vi "SwerveOdometry_UpdateX.vi"(8 "module Positions":T6[](array[typedef]) {"Angle"."SIN" format="%13.4f"; "Angle"."COS" format="%13.4f"; "Angle"."VALUE" format="%13.4f"}, 9 "gyroAngle":T5={"VALUE"=0.0, "COS"=1.0, "SIN"=0.0} {"SIN" format="%13.4f"; "COS" format="%13.4f"; "VALUE" format="%13.4f"}, 10 "in SWERVE_DRIVE_ODOMETRY":T8={"POSE"={"TRANSLATION"={"X"=0.0, "Y"=0.0}, "ROTATION"={"VALUE"=0.0, "COS"=1.0, "SIN"=0.0}}, "GyroOffset"={"VALUE"=0.0, "COS"=1.0, "SIN"=0.0}, "PreviousAngle"={"VALUE"=0.0, "COS"=1.0, "SIN"=0.0}, "PrevModulePositions"=[], "NumModules"=0} {"PrevModulePositions"."Angle"."SIN" format="%13.4f"; "PrevModulePositions"."Angle"."COS" format="%13.4f"; "PrevModulePositions"."Angle"."VALUE" format="%13.4f"; "PreviousAngle"."SIN" format="%13.4f"; "PreviousAngle"."COS" format="%13.4f"; "PreviousAngle"."VALUE" format="%13.4f"; "GyroOffset"."SIN" format="%13.4f"; "GyroOffset"."COS" format="%13.4f"; "GyroOffset"."VALUE" format="%13.4f"; "POSE"."ROTATION"."SIN" format="%13.4f"; "POSE"."ROTATION"."COS" format="%13.4f"; "POSE"."ROTATION"."VALUE" format="%13.4f"; "POSE"."TRANSLATION"."Y" format="%14.3f"; "POSE"."TRANSLATION"."X" format="%14.3f"}, 11 "SWERVE_DRIVE_KINEMATICS":T1 {"SavedModuleStates"."Angle"."SIN" format="%13.4f"; "SavedModuleStates"."Angle"."COS" format="%13.4f"; "SavedModuleStates"."Angle"."VALUE" format="%13.4f"; "PrevCoR"."Y" format="%14.3f"; "PrevCoR"."X" format="%14.3f"; "Modules"."Y" format="%14.3f"; "Modules"."X" format="%14.3f"}) -> (0 "Error":bool, 1 "robot POSE":T7={"TRANSLATION"={"X"=0.0, "Y"=0.0}, "ROTATION"={"VALUE"=0.0, "COS"=1.0, "SIN"=0.0}} {"ROTATION"."SIN" format="%13.4f"; "ROTATION"."COS" format="%13.4f"; "ROTATION"."VALUE" format="%13.4f"; "TRANSLATION"."Y" format="%14.3f"; "TRANSLATION"."X" format="%14.3f"}, 3 "out SWERVE_DRIVE_ODOMETRY":T8={"POSE"={"TRANSLATION"={"X"=0.0, "Y"=0.0}, "ROTATION"={"VALUE"=0.0, "COS"=1.0, "SIN"=0.0}}, "GyroOffset"={"VALUE"=0.0, "COS"=1.0, "SIN"=0.0}, "PreviousAngle"={"VALUE"=0.0, "COS"=1.0, "SIN"=0.0}, "PrevModulePositions"=[], "NumModules"=0} {"PrevModulePositions"."Angle"."SIN" format="%13.4f"; "PrevModulePositions"."Angle"."COS" format="%13.4f"; "PrevModulePositions"."Angle"."VALUE" format="%13.4f"; "PreviousAngle"."SIN" format="%13.4f"; "PreviousAngle"."COS" format="%13.4f"; "PreviousAngle"."VALUE" format="%13.4f"; "GyroOffset"."SIN" format="%13.4f"; "GyroOffset"."COS" format="%13.4f"; "GyroOffset"."VALUE" format="%13.4f"; "POSE"."ROTATION"."SIN" format="%13.4f"; "POSE"."ROTATION"."COS" format="%13.4f"; "POSE"."ROTATION"."VALUE" format="%13.4f"; "POSE"."TRANSLATION"."Y" format="%14.3f"; "POSE"."TRANSLATION"."X" format="%14.3f"})   [LabVIEW 2019, in "Trajectory_Library.lvlib"]
doc: "Updates the robot's position on the field using forward kinematics and integration of the pose over time. This method takes in the current time as a parameter to calculate period (difference between two timestamps). The period is used to calculate the change in distance from a velocity. Thisalso takes in an angle parameter which is used instead of the angular rate that is calculated from forward kinematics.\n\nParameters:\n - InSwerveDriveKinematics - The data structure \n - InSwerveDriveOdometry - This data structure \n - gyroAngle - The angle reported by the gyroscope.\n - modulePositions - The current positions (distances) of all swerve modules. Please provide the states in the same order in which you instantiated your SwerveDriveKinematics.\n\nReturns:\n - OutSwerveDriveOdometry - Updated data structure\n - The new pose of the robot.\n - Error -- TRUE if an error occured (number of modules doesn't match)"
uses:
  Trajectory_Library.lvlib
  TypeDef/TRANSLATION2D.ctl
  TypeDef/ROTATION2D.ctl
  TypeDef/POSE2D.ctl
  TypeDef/SWERVE_DRIVE_ODOMETRY.ctl
  TypeDef/SWERVE_DRIVE_MODULE_STATE.ctl
  <vilib>/Analysis/Matrix/Datatypes/RealMatrix.ctl
  <vilib>/Analysis/Matrix/NI_Matrix.lvlib
  TypeDef/SWERVE_DRIVE_KINEMATICS.ctl
  TypeDef/SWERVE_DRIVE_MODULE_POSITION.ctl
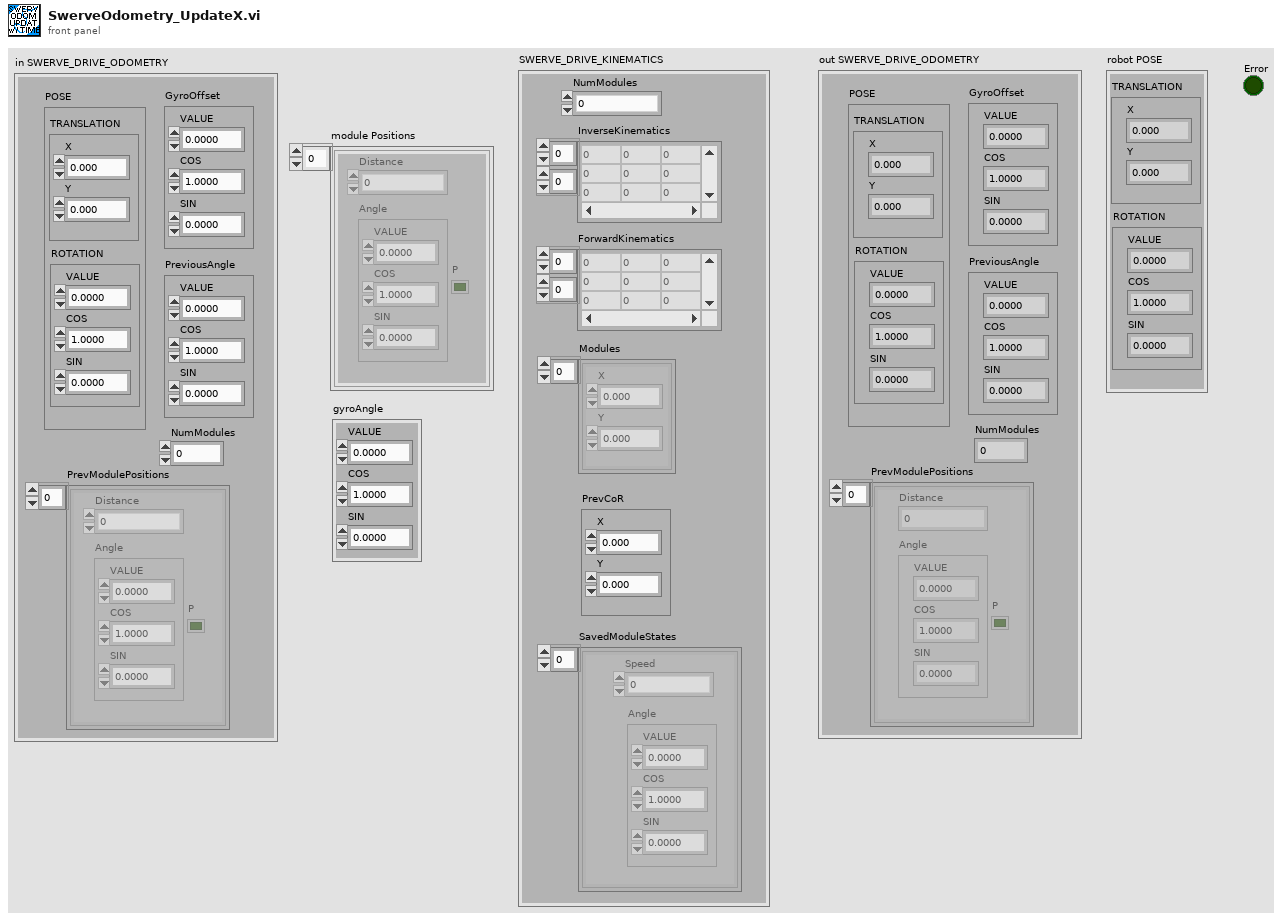
[diagram p1: front panel]
types:
  T1 = typedef "Trajectory_Library.lvlib/SWERVE_DRIVE_KINEMATICS.ctl" = cluster{"NumModules":i32, "InverseKinematics":T2, "ForwardKinematics":T2, "Modules":T3[], "PrevCoR":T3, "SavedModuleStates":T4[]}
  T2 = typedef "NI_Matrix.lvlib/RealMatrix.ctl" = dbl[][]
  T3 = typedef "Trajectory_Library.lvlib/TRANSLATION2D.ctl" = cluster{"X":dbl, "Y":dbl}
  T4 = typedef "Trajectory_Library.lvlib/SWERVE_DRIVE_MODULE_STATE.ctl" = cluster{"Speed":dbl, "Angle":T5}
  T5 = typedef "Trajectory_Library.lvlib/ROTATION2D.ctl" = cluster{"VALUE":dbl, "COS":dbl, "SIN":dbl}
  T6 = typedef "Trajectory_Library.lvlib/SWERVE_DRIVE_MODULE_POSITION.ctl" = cluster{"Distance":dbl, "Angle":T5, "P":bool}
  T7 = typedef "Trajectory_Library.lvlib/POSE2D.ctl" = cluster{"TRANSLATION":T3, "ROTATION":T5}
  T8 = typedef "Trajectory_Library.lvlib/SWERVE_DRIVE_ODOMETRY.ctl" = cluster{"POSE":T7, "GyroOffset":T5, "PreviousAngle":T5, "PrevModulePositions":T6[], "NumModules":i32}
  T9 = typedef "Trajectory_Library.lvlib/TWIST2D.ctl" = cluster{"dX":dbl, "dY":dbl, "dTHETA":dbl}
  T10 = typedef "WPILib_Math.lvlib/POSE2D.ctl" = cluster{"TRANSLATION":T11, "ROTATION":T12}
  T11 = typedef "WPILib_Math.lvlib/TRANSLATION2D.ctl" = cluster{"X":dbl, "Y":dbl}
  T12 = typedef "WPILib_Math.lvlib/ROTATION2D.ctl" = cluster{"VALUE":dbl, "COS":dbl, "SIN":dbl}
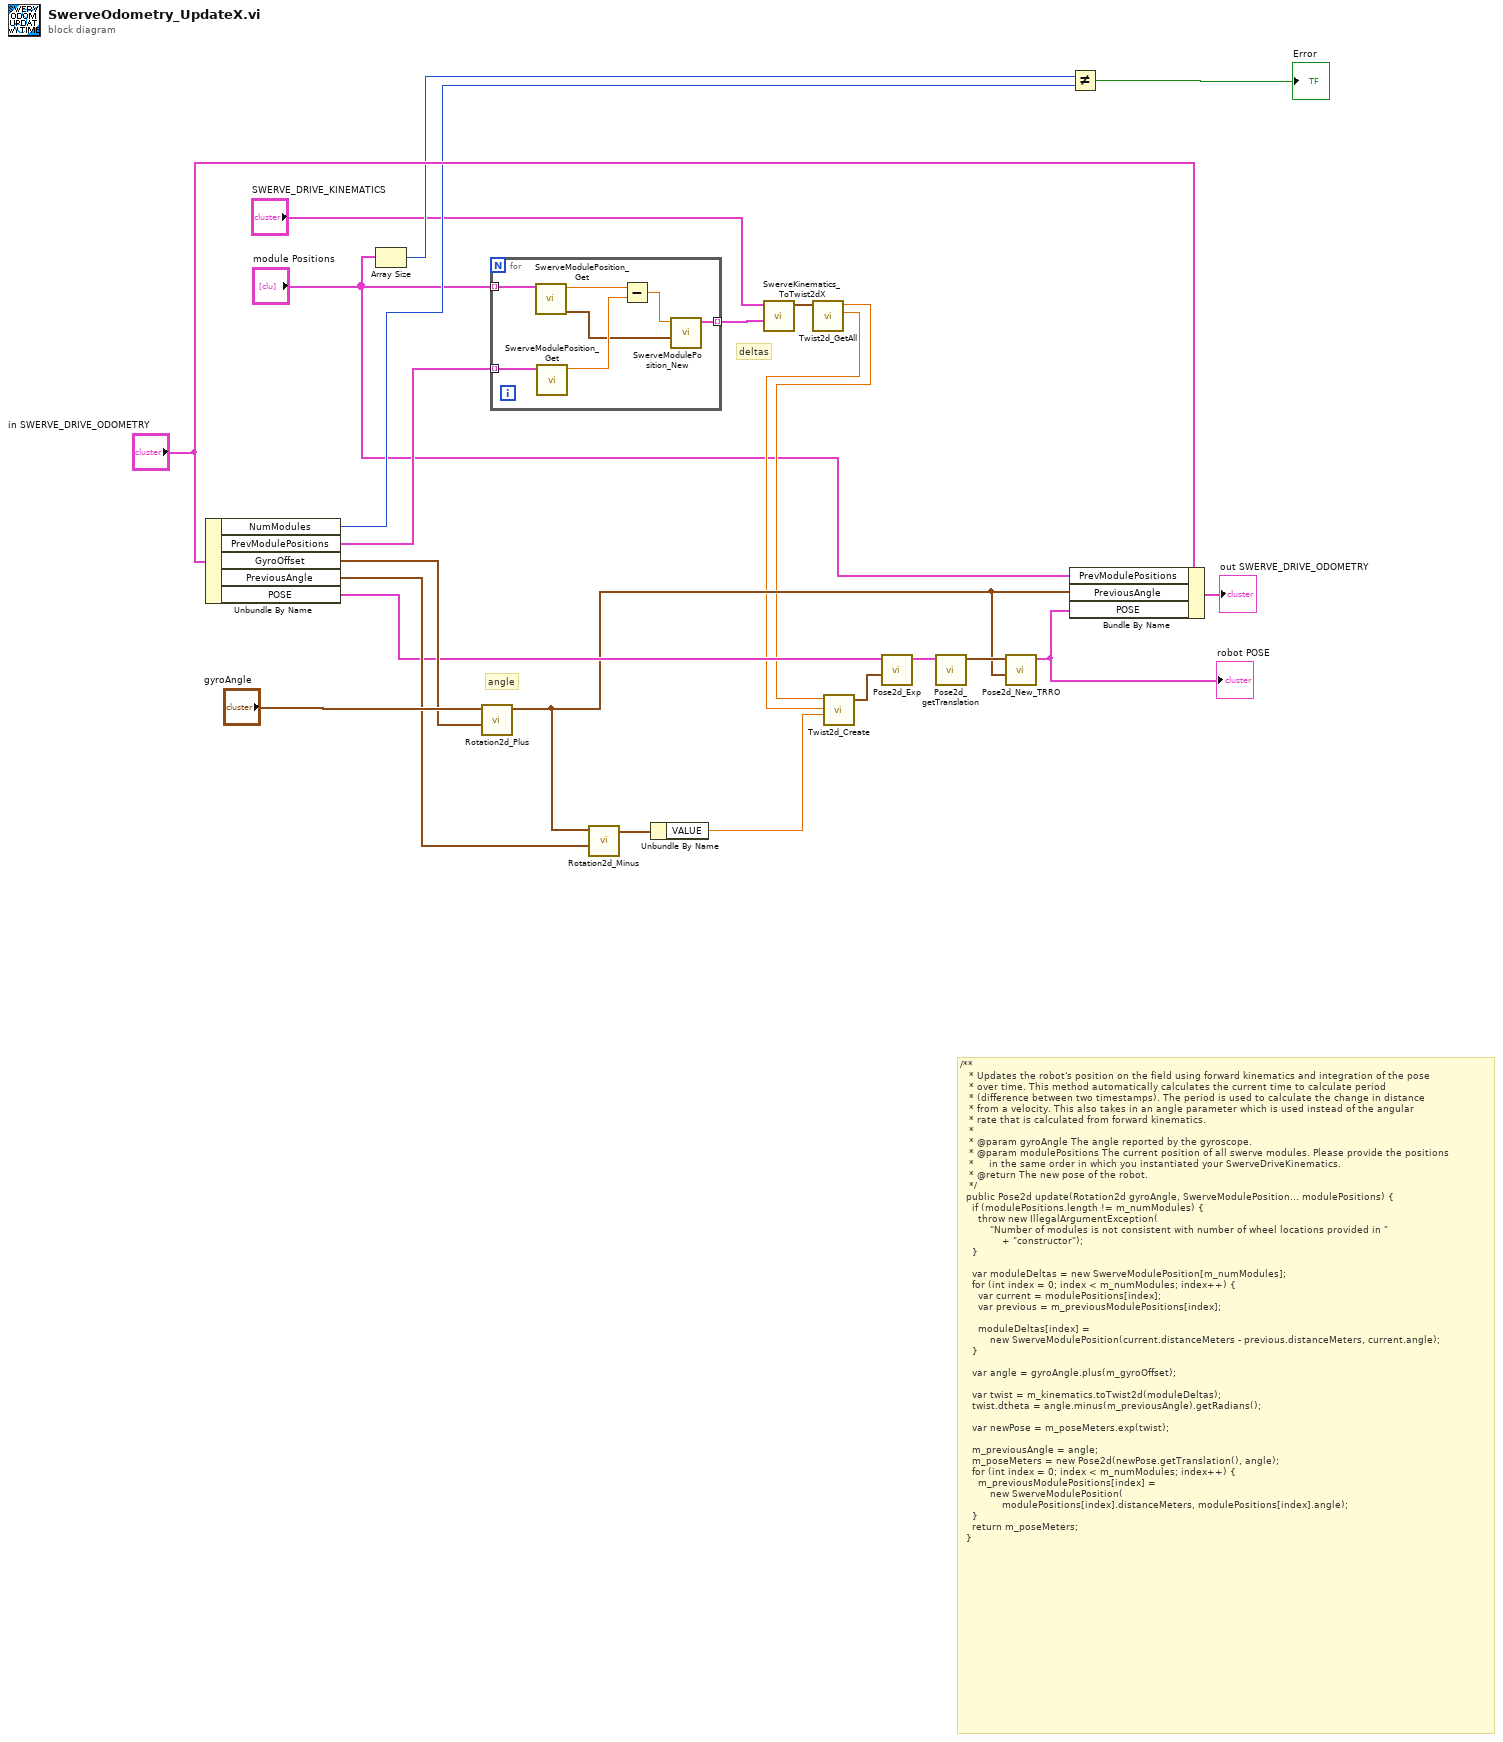
[diagram p0: block diagram]
diagram:
  # "deltas"
  # "/**\n   * Updates the robot's position on the field using forward kinematics and integration of the pose\n   * over time. This method automatically calculates the current time to calculate period\n   * (difference between two timestamps). The period is used to calculate the change in distance\n   * from a velocity. This also takes in an angle parameter which is used instead of the angular\n   * rate that is calculated from forward kinematics.\n   *\n   * @param gyroAngle The angle reported by the gyroscope.\n   * @param modulePositions The current position of all swerve modules. Please provide the positions\n   *     in the same order in which you instantiated your SwerveDriveKinematics.\n   * @return The new pose of the robot.\n   */\n  public Pose2d update(Rotation2d gyroAngle, SwerveModulePosition... modulePositions) {\n    if (modulePositions.length != m_numModules) {\n      throw new IllegalArgumentException(\n          \"Number of modules is not consistent with number of wheel locations provided in \"\n              + \"constructor\");\n    }\n\n    var moduleDeltas = new SwerveModulePosition[m_numModules];\n    for (int index = 0; index < m_numModules; index++) {\n      var current = modulePositions[index];\n      var previous = m_previousModulePositions[index];\n\n      moduleDeltas[index] =\n          new SwerveModulePosition(current.distanceMeters - previous.distanceMeters, current.angle);\n    }\n\n    var angle = gyroAngle.plus(m_gyroOffset);\n\n    var twist = m_kinematics.toTwist2d(moduleDeltas);\n    twist.dtheta = angle.minus(m_previousAngle).getRadians();\n\n    var newPose = m_poseMeters.exp(twist);\n\n    m_previousAngle = angle;\n    m_poseMeters = new Pose2d(newPose.getTranslation(), angle);\n    for (int index = 0; index < m_numModules; index++) {\n      m_previousModulePositions[index] =\n          new SwerveModulePosition(\n              modulePositions[index].distanceMeters, modulePositions[index].angle);\n    }\n    return m_poseMeters;\n  }"
  # "angle"
  n1 = Unbundle By Name("in SWERVE_DRIVE_ODOMETRY") -> ("NumModules"=w8:i32, "PrevModulePositions"=w10:T6[], "GyroOffset"=w20:T5, "PreviousAngle"=w19:T5, "POSE"=w16:T7)
  n2 = Array Size(array="module Positions") -> (size(s)=w9:i32)
  n3 = call "Rotation2d_Plus.vi"("other ROTATION"=w20, "in ROTATION"="gyroAngle") -> ("out ROTATION"=w12:T5)  [unwired: 9 in]
  n4 = for {
    tunnel: w10 -> [w30] mode=indexing
    tunnel: "module Positions" -> [w29] mode=indexing
    tunnel: [w24] -> w5 mode=indexing
    n5 = call "SwerveModulePosition_Get.vi"("Swerve Module Position"=w29) -> ("Angle Rotation2d"=w25:T5, "Distance M"=w28:dbl)  [unwired: 8 in, 1 out]
    n6 = call "SwerveModulePosition_Get.vi"("Swerve Module Position"=w30) -> ("Distance M"=w27:dbl)  [unwired: 8 in, 2 out]
    n7 = Subtract(x=w28, y=w27) -> (x-y=w26:dbl)
    n8 = call "SwerveModulePosition_New.vi"("ROTATION"=w25, "Distance"=w26) -> ("SWERVE_DRIVE_MODULE_POSITION"=w24:T6)  [unwired: 9 in]
  }
  n9 = call "Rotation2d_Minus.vi"("other ROTATION"=w19, "in ROTATION"=w12) -> ("out ROTATION"=w18:T5)  [unwired: 9 in]
  n10 = Unbundle By Name(w18) -> ("VALUE"=w17:dbl)
  n11 = call "SwerveKinematics_ToTwist2dX.vi"("WheelDeltas"=w5, "in SWERVE_DRIVE_KINEMATICS"="SWERVE_DRIVE_KINEMATICS") -> ("Twist2d"=w4:T9)  [unwired: 8 in, 1 out]
  n12 = call "Twist2d_GetAll.vi"("TWIST"=w4) -> ("dY"=w2:dbl, "dX"=w3:dbl)  [unwired: 8 in, 1 out]
  n13 = call "Twist2d_Create.vi"("dTHETA"=w17, "dY"=w2, "dX"=w3) -> ("TWIST"=w15:T9)  [unwired: 8 in]
  n14 = call "Pose2d_Exp.vi"("TWIST"=w15, "POSE"=w16) -> ("UpdatedPose"=w14:T10)  [unwired: 9 in]
  n15 = call "Pose2d_getTranslation.vi"("in POSE"=w14) -> ("outTRANSLATION"=w13:T3)  [unwired: 10 in]
  n16 = call "Pose2d_New_TRRO.vi"("ROTATION"=w12, "TRANSLATION"=w13) -> ("outPOSE"=w11:T7)  [unwired: 9 in]
  "robot POSE" <- w11
  n17 = Not Equal?(x=w9, y=w8) -> (x != y?=→"Error":bool)
  n18 = Bundle By Name(cluster="in SWERVE_DRIVE_ODOMETRY", "PrevModulePositions"="module Positions", "PreviousAngle"=w12, "POSE"=w11) -> (→"out SWERVE_DRIVE_ODOMETRY":T8)
